vi "conversion_m_to_cm.vi"(1 "x (m)":dbl) -> (0 "x (cm)":dbl)   [LabVIEW 2021]
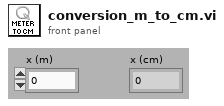
[diagram p1: front panel]
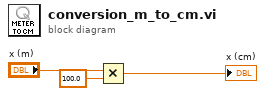
[diagram p0: block diagram]
diagram:
  n1 = Multiply(x="x (m)", y=100.0) -> (x*y=→"x (cm)":dbl)
